vi "Ex 01 - Simple A-Scan.vi"() -> ()   [LabVIEW 2026]
uses:
  <instrlib>/MicroPulse/Public/Data/Datatypes/MP - data formatting.ctl
  <instrlib>/MicroPulse/Public/Data/Datatypes/MP - amplitude reporting mode.ctl
  <instrlib>/MicroPulse/Public/Data/Datatypes/MP - averaging.ctl
  <instrlib>/MicroPulse/Public/Data/Datatypes/MP - transmit parameters.ctl
  <instrlib>/MicroPulse/Public/Data/Datatypes/MP - pulser voltage.ctl
  <instrlib>/MicroPulse/Public/Data/Datatypes/MP - pulse damping.ctl
  <instrlib>/MicroPulse/Public/Data/Datatypes/MP - test parameters.ctl
  <instrlib>/MicroPulse/Public/Data/Datatypes/MP - receive parameters.ctl
  Public/Data/Datatypes/MP - display gate.ctl
  <instrlib>/MicroPulse/Public/Data/Datatypes/MP - waveform type.ctl
  <instrlib>/MicroPulse/Public/Data/Datatypes/MP - analogue filter.ctl
  <instrlib>/MicroPulse/Public/Data/Datatypes/MP - frequency filter.ctl
  <instrlib>/MicroPulse/Public/Data/Datatypes/MP - digital filtering.ctl
  <instrlib>/MicroPulse/Public/Data/Datatypes/MP - high pass filter.ctl
  <instrlib>/MicroPulse/Public/Data/Datatypes/MP - low pass filter.ctl
  Public/Data/Datatypes/TCP config.ctl
  Public/Data/Datatypes/MP - sample frequency.ctl
  <instrlib>/MicroPulse/Public/Data/Datatypes/MP - instrument type.ctl
  Public/Data/Datatypes/MP - echo gate mode.ctl
  MicroPulse_Driver.lvlib
  <vilib>/ptbypt/NI_PtbyPt.lvlib
panel:
  out "Instrument Type":T1
  out "Sample Frequency":T2
  out "Command List":string
  in  "stop":bool
  out "running average PRF":dbl format="%0.2f"
  out "AScan Graph":u16[](graph)
  out "error out":errorcluster
  out "message count":i32
  out "System Messages":string
  in  "TCP config":T3={"Connection ID"=refnum, "IP address"="10.1.1.2", "host port"=1067, "OC timeout"=5000, "Read timeout"=100, "Write timeout"=100} {"Write timeout" format="%dms"; "Read timeout" format="%dms"; "OC timeout" format="%dms"}
  in  "Receive Parameters":T4={"Display Gate"={"Start"=0.0, "Length"=100.0}, "Delay"=0.0, "Waveform Type"=enum."Rectified Signal", "Gain"=0.0, "Analogue Filtering"={"Bandpass"=enum."No change", "Smoothing"=1}, "Digital Filtering"={"High Pass Filter"=enum."None", "Low Pass Filter"=enum."None"}} {"Delay" format="%#_g us"; "Display Gate"."Length" min=0.0 max=64000.0 step=1000.0 format="%#_g us"; "Display Gate"."Start" min=0.0 max=64000.0 step=1000.0 format="%#_g us"; "Analogue Filtering"."Smoothing" min=1 max=11 step=1; "Gain" min=-6.0 max=70.0 step=0.25 format="%.2fdB"}
  in  "Test Parameters":T12={"Test No."=1, "Tx Channel"=1, "Rx Channel"=1} {"Rx Channel" min=1 max=1024; "Tx Channel" min=1 max=1024}
  in  "Transmit Parameters":T13={"Pulse Voltage"=enum."50V", "Pulse Shape"={"Damping"=enum."660W", "Width"=250}} {"Pulse Shape"."Width" min=16 max=1010 step=50 format="%.0fns"}
  in  "Data Formatting":T16={"Amplitude Mode"=enum."Ascan Data", "Averaging"=enum."None", "Coupling Level"=0} {"Coupling Level" max=4095 step=1}
  # "Example 01 - Simple A-scan Test\n\nSet all controls to the required values\nbefore running the VI.\n\nWhile running, test parameters may not be changed.\n\nThis example uses the instrument's default values for Data Output Format, Pulse Repetition Frequency and Sampling Rate."
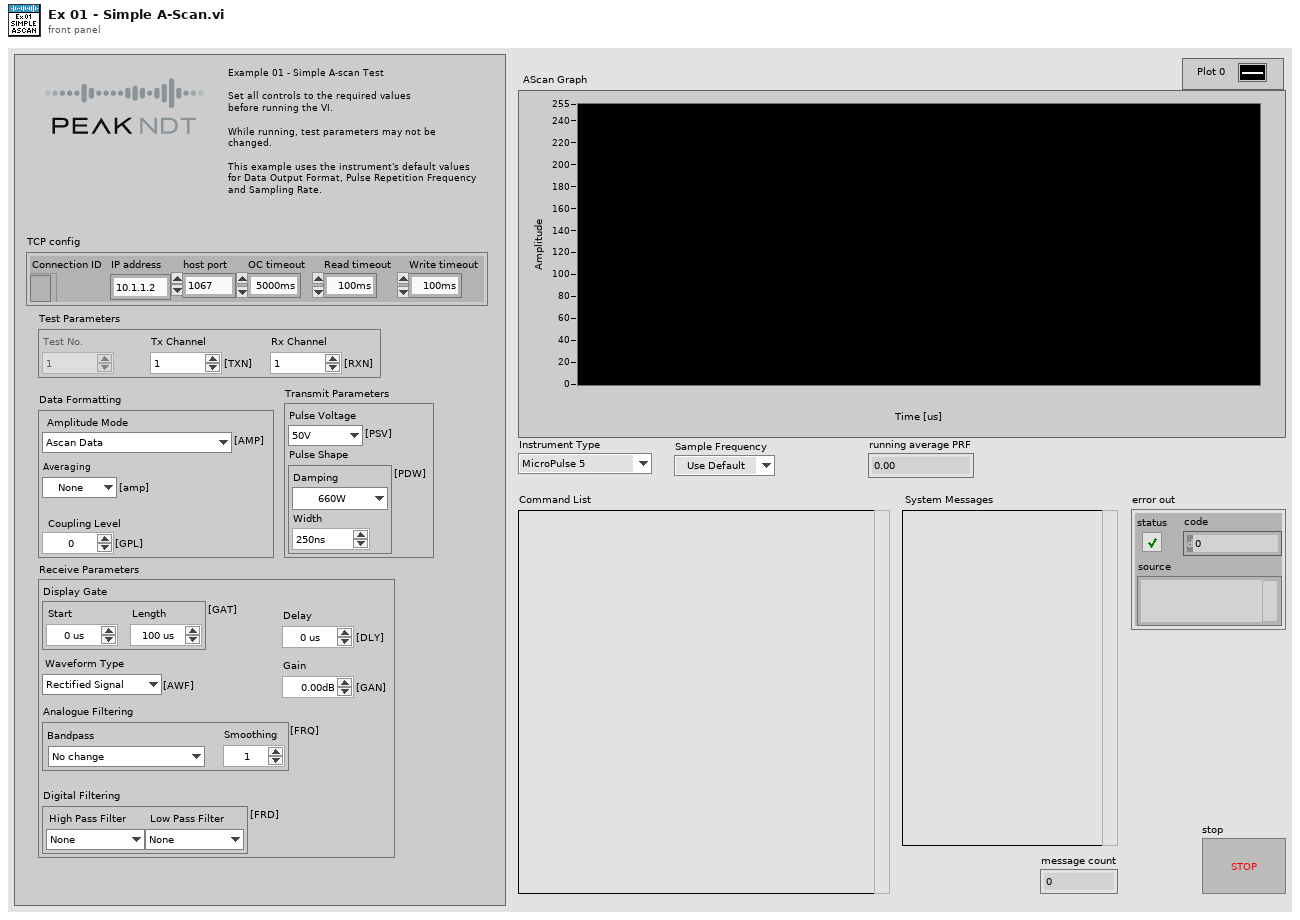
[diagram p1: front panel]
types:
  T1 = typedef "MicroPulse_Driver.lvlib/MP - instrument type.ctl" = enum16{"MicroPulse 5", "LT1", "LT2", "LTPA", "MPLT", "MicroPulse 6", "PipeScanner", "<MicroPulse>", "Micropulse 4", "Simulated Data"}
  T2 = typedef "MicroPulse_Driver.lvlib/MP - sample frequency.ctl" = enum16{"Use Default", "200MHz (LT2 only)", "100MHz", "50MHz", "25MHz", "10MHz"}
  T3 = typedef "MicroPulse_Driver.lvlib/TCP config.ctl" = cluster{"Connection ID":refnum<k5>, "IP address":string, "host port":u16, "OC timeout":i32, "Read timeout":i32, "Write timeout":i32}
  T4 = typedef "MicroPulse_Driver.lvlib/MP - receive parameters.ctl" = cluster{"Display Gate":T5, "Delay":dbl, "Waveform Type":T6, "Gain":dbl, "Analogue Filtering":T7, "Digital Filtering":T9}
  T5 = typedef "MicroPulse_Driver.lvlib/MP - display gate.ctl" = cluster{"Start":dbl, "Length":dbl}
  T6 = typedef "MicroPulse_Driver.lvlib/MP - waveform type.ctl" = enum16{"Rectified Signal", "RF Signal", "+Half Wave", "-Half Wave"}
  T7 = typedef "MicroPulse_Driver.lvlib/MP - analogue filter.ctl" = cluster{"Bandpass":T8, "Smoothing":u16}
  T8 = typedef "MicroPulse_Driver.lvlib/MP - frequency filter.ctl" = enum16{"No change", "1MHz Bandpass", "2MHz Bandpass", "4MHz Bandpass", "5MHz Bandpass", "10MHz Bandpass", "2.5-18MHz Broadband", "0.75-12MHz  Broadband", "0.5MHz Bandpass", "5MHz 2nd Order TOFD", "10MHz 2nd Order TOFD", "3.0-25MHz Broadband", "3.0-30MHz Broadband"}
  T9 = typedef "MicroPulse_Driver.lvlib/MP - digital filtering.ctl" = cluster{"High Pass Filter":T10, "Low Pass Filter":T11}
  T10 = typedef "MicroPulse_Driver.lvlib/MP - high pass filter.ctl" = enum16{"None", "0.7MHz", "1.5MHz", "4.0MHz", "7.5MHz", "10.0MHz", "User Defined"}
  T11 = typedef "MicroPulse_Driver.lvlib/MP - low pass filter.ctl" = enum16{"None", "1.8MHz", "3.0MHz", "6.0MHz", "8.0MHz", "12.0MHz", "User Defined"}
  T12 = typedef "MicroPulse_Driver.lvlib/MP - test parameters.ctl" = cluster{"Test No.":u32, "Tx Channel":u32, "Rx Channel":u32}
  T13 = typedef "MicroPulse_Driver.lvlib/MP - transmit parameters.ctl" = cluster{"Pulse Voltage":T14, "Pulse Shape":cluster{"Damping":T15, "Width":u32}}
  T14 = typedef "MicroPulse_Driver.lvlib/MP - pulser voltage.ctl" = enum16{"50V", "100V", "150V", "200V", "250V", "300V"}
  T15 = typedef "MicroPulse_Driver.lvlib/MP - pulse damping.ctl" = enum16{"660W", "458W", "220W", "149W", "102W", "82W", "63W", "51W"}
  T16 = typedef "MicroPulse_Driver.lvlib/MP - data formatting.ctl" = cluster{"Amplitude Mode":T17, "Averaging":T18, "Coupling Level":u32}
  T17 = typedef "MicroPulse_Driver.lvlib/MP - amplitude reporting mode.ctl" = enum16{"1st Peak in gate", "Maximum Peak in gate", "All Peaks", "Ascan Data", "1st Threshold Crossing Peak", "Ascan + Peaks", "All Peaks for Multigate", "Peaks + Ascan for Multigate", "Peaks + P_Ascan for Multigate", "Full Matrix Capture"}
  T18 = typedef "MicroPulse_Driver.lvlib/MP - averaging.ctl" = enum16{"None", "2", "4", "8", "16", "32", "64", "128", "256"}
  T19 = typedef "MicroPulse_Driver.lvlib/MP - echo gate mode.ctl" = enum16{"Echo Trigger OFF", "Echo Gate Display Mode", "Echo Trigger ON", "Multi Gate or FMC Mode", "Reserved", "PA - Echo Trigger ON"}
  T20 = typedef "MicroPulse_Driver.lvlib/MP-Registry Data-Cluster.ctl" = cluster{"Instrument Type":T1, "Serial #":u64, "Sample Frequency":T2, "dt (us)":dbl, "DOF":T21, "Material Velocity":dbl, "Asynch Reads":T22, "NUM of Tests":u32, "System Details":T23, "Gates":T25[], "Encoders":T30[], "CMD LUT":variant, "Command List":string}
  T21 = typedef "MicroPulse_Driver.lvlib/MP - data output format.ctl" = enum16{"", "8-bit Mode", "10-bit Mode", "12-bit Mode", "16-bit Mode", "8-bit Log Mode", "12-bit Packed Mode"}
  T22 = typedef "MicroPulse_Driver.lvlib/MP - asynch read mode.ctl" = enum16{"Disabled", "Enabled"}
  T23 = typedef "MicroPulse_Driver.lvlib/MP - general system status.ctl" = cluster{"System Type":T1, "Serial No.":u64, "Channels":cluster{"Conv":u8, "PA":u16, "Extra":u32}, "Sample Frequency":cluster{"Default":u8, "Actual":u8}, "Software Versions":string, "Data Output Format":cluster{"Default":T21, "Actual":T21}, "Temperatures":cluster{"System":u8, "Processor":u8, "Slave Sys":u8, "Slave Proc":u8}, "Tx Buffer Size":u32, "System Error":string, "No. of Cards":u8, "DAC Gain":i16, "Uptimes":cluster{"since Power":u32, "since RSTS":u32, "since SRST":u32}, "Voltages":cluster{"Nominal":dbl, "Measured":dbl, "Difference":dbl}[], "Interface Cards":T24[]}
  T24 = typedef "MicroPulse_Driver.lvlib/MP - interface card status.ctl" = cluster{"Status":u8, "Map":u8, "Board - T":u8, "FPGA - T":u8, "PAIF Status":string, "Version":string}
  T25 = typedef "MicroPulse_Driver.lvlib/MP - Registry Gates.ctl" = cluster{"Display Gate":T5, "ETM Mode":T19, "Echo Gate":T26, "Insp Gates":T27[]}
  T26 = typedef "MicroPulse_Driver.lvlib/MP - echo gate parameters.ctl" = cluster{"Start (us)":dbl, "Length (us)":dbl, "Threshold":u16, "Colour":u32}
  T27 = typedef "MicroPulse_Driver.lvlib/MP - multigate inspection gate parameters.ctl" = cluster{"Start (us)":dbl, "Length (us)":dbl, "Threshold":u16, "Enabled?":bool, "Max # Peaks":u16, "Hysteresis":T28, "Mode":T29, "Inverted?":bool, "Colour ":u32}
  T28 = typedef "MicroPulse_Driver.lvlib/MP - hysteresis level.ctl" = enum16{"None", "3dB", "6dB", "9dB", "12dB"}
  T29 = typedef "MicroPulse_Driver.lvlib/MP - multigate mode.ctl" = enum16{"1st Peak in Gate", "Largest Peak In Gate", "All Peaks In Gate", "1st Threshold Crossing"}
  T30 = typedef "MicroPulse_Driver.lvlib/MP - encoder settings.ctl" = cluster{"Encoder Type":T31, "Counts/mm":u32, "Enable Termination?":bool, "Multiplier":u32, "Backlash Period (s)":dbl, "Encoder Filter":u32}
  T31 = typedef "MicroPulse_Driver.lvlib/MP - encoder type.ctl" = enum16{"Quadrature", "Step/Direction"}
  T32 = typedef "MicroPulse_Driver.lvlib/MP - scan data info.ctl" = cluster{"Message Header":u16, "Error Message":u16, "Test No.":u32, "Channel No.":u8, "Sweep No.":u32, "Gate No.":u32, "DOF":T21, "retain data":T33, "scan data":u16[], "scan length":i32, "scan index":i32, "peak data":cluster{"timebase":u16[], "data":u16[]}, "#peaks":i32, "PRF":dbl, "IP":cluster{"Axis No.":u8, "Location":u32, "MIP location":u32, "MIP?":bool}, "echo range":u16, "ETG":bool, "CAL 0 complete":bool, "Axis Positions":T34}
  T33 = typedef "MicroPulse_Driver.lvlib/MP - retain scan.ctl" = enum16{"None", "Ascan", "Peaks"}
  T34 = typedef "MicroPulse_Driver.lvlib/MP - axis positions (LLC).ctl" = cluster{"Axis 1":u32, "Axis 2":u32, "Axis 3":u32, "Axis 4":u32, "Status":u8}
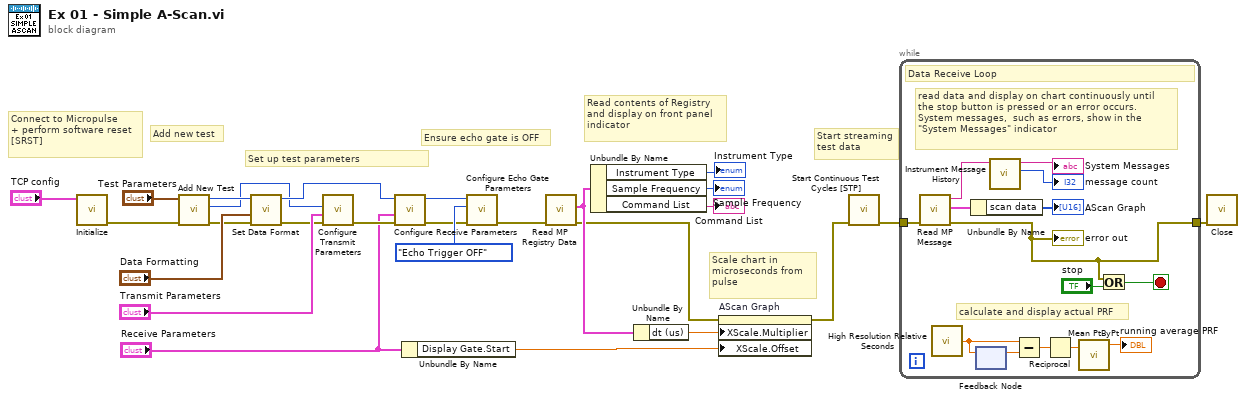
[diagram p0: block diagram]
diagram:
  # "Scale chart in \nmicroseconds from\npulse"
  # "Start streaming\ntest data"
  # "Set up test parameters"
  # "Connect to Micropulse\n+ perform software reset\n[SRST]"
  # "Add new test"
  # "Ensure echo gate is OFF"
  # "Read contents of Registry\nand display on front panel\nindicator"
  n1 = call "Initialize.vi"("TCP config"="TCP config") -> ("error out"=w21:errorcluster)  [unwired: 9 in, 1 out]
  n2 = call "Add New Test.vi"("error in (no error)"=w21, "Test Parameters"="Test Parameters") -> ("error out"=w18:errorcluster, "Tx Channel out"=w7:u32, "Test No. out"=w10:u32)  [unwired: 6 in, 1 out]
  n3 = call "Set Data Format.vi"("error in (no error)"=w18, "Data Formatting"="Data Formatting", "Test No."=w10) -> ("error out"=w17:errorcluster, "Test No. out"=w9:u32)  [unwired: 6 in, 1 out]
  n4 = call "Configure Transmit Parameters.vi"("error in (no error)"=w17, "Transmit Parameters"="Transmit Parameters", "Tx Channel"=w7) -> ("error out"=w22:errorcluster)  [unwired: 7 in, 1 out]
  n5 = call "Configure Receive Parameters.vi"("error in (no error)"=w22, "Receive Parameters"="Receive Parameters", "Test No."=w9) -> ("error out"=w16:errorcluster, "Test No. out"=w8:u32)  [unwired: 6 in, 1 out]
  n6 = Unbundle By Name("Receive Parameters") -> ("Display Gate.Start"=w11:dbl)
  n7 = call "Configure Echo Gate Parameters.vi"("error in (no error)"=w16, "Echo Trigger Mode"=MP_-_echo_gate_mode."Echo Trigger OFF" ("ETM Mode"), "Test Number"=w8) -> ("error out"=w20:errorcluster)  [unwired: 6 in, 2 out]
  n8 = call "Read MP Registry Data.vi"("error in (no error)"=w20) -> ("error out"=w5:errorcluster, "Micropulse Data"=w14:T20)  [unwired: 7 in, 2 out]
  n9 = Unbundle By Name(w14) -> ("Instrument Type"=→"Instrument Type":T1, "Sample Frequency"=→"Sample Frequency":T2, "Command List"=→"Command List":string)
  n10 = Unbundle By Name(w14) -> ("dt (us)"=w13:dbl)
  n11 = property on="AScan Graph" class="WFGraph (strict)"(error in=w5, "XScale.Multiplier"=w13, "XScale.Offset"=w11) -> (error out=w4:errorcluster)  [unwired: 1 in, 1 out]
  n12 = call "Start Continuous Test Cycles [STP].vi"("error in (no error)"=w4) -> ("error out"=w6:errorcluster)  [unwired: 9 in, 1 out]
  n13 = while {
    tunnel: [w29] -> w15
    tunnel: w6 -> [w27]
    stop <- w40 stop-if-true
    # "calculate and display actual PRF"
    # "read data and display on chart continuously until\nthe stop button is pressed or an error occurs.\nSystem messages,  such as errors, show in the \n\"System Messages\" indicator"
    # "Data Receive Loop"
    n14 = call "Read MP Message.vi"("error in (no error)"=w27) -> ("error out"=w29:errorcluster, "scan data info"=w39:T32, "Instrument Message"=w32:string)  [unwired: 6 in, 2 out]
    "error out" <- w29
    n15 = call <vilib>:"High Resolution Relative Seconds.vi"() -> ("relative seconds"=w37:dbl)
    n16 = Unbundle By Name(w39) -> ("scan data"=→"AScan Graph":u16[])
    n17 = feedback-in #1(w37) -> ()
    n18 = feedback #1() -> (w36:dbl)  [unwired: 1 in]
    n19 = call "Instrument Message History.vi"("Instrument Message"=w32) -> ("Message Count"=→"message count":i32, "Message History out"=→"System Messages":string)  [unwired: 9 in]
    n20 = Subtract(x=w37, y=w36) -> (x-y=w35:dbl)
    n21 = Reciprocal(x=w35) -> (1/x=w34:dbl)
    n22 = call <vilib>:"Mean PtByPt.vi"("x"=w34) -> ("mean"=→"running average PRF":dbl)  [unwired: 3 in, 1 out]
    n23 = Or(x=w29, y="stop") -> (x .or. y?=w40:bool)
  }
  n24 = call "Close.vi"("error in (no error)"=w15) -> ()  [unwired: 9 in, 2 out]
